vi "SeCrTs-UI Commands_R.vi"(11 "Data FIFO Ref":T1) -> ()   [LabVIEW 2022 SP3]
doc: "Use this template to build a simple state machine design pattern. Each state executes code and determines which state to transition to."
uses:
  RT Controls/SeCrTs-Data FIFO.ctl
  RT Controls/SeCrTs-NS Enum.ctl
  RT Controls/SeCrTs-Data Type Control screen.ctl
  RT Support/SeCrTs-RT_Global_R.vi
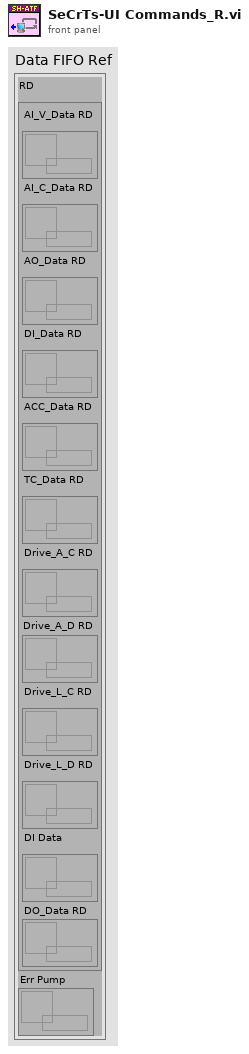
[diagram p1: front panel]
types:
  T1 = typedef "SeCrTs-Data FIFO.ctl" = cluster{"RD":cluster{"AI_V_Data RD":refnum<queue>, "AI_C_Data RD":refnum<queue>, "AO_Data RD":refnum<queue>, "DI_Data RD":refnum<queue>, "ACC_Data RD":refnum<queue>, "TC_Data RD":refnum<queue>, "Drive_A_C RD":refnum<queue>, "Drive_A_D RD":refnum<queue>, "Drive_L_C RD":refnum<queue>, "Drive_L_D RD":refnum<queue>, "DI Data":refnum<queue>, "DO_Data RD":refnum<queue>}, "Err Pump":refnum<queue>}
  T2 = typedef "SeCrTs-Data Type Control screen.ctl" = cluster{"DI_Data":digitalwaveform[], "Drive_A_C":waveform(dbl)[], "Drive_A_D":waveform(dbl)[], "Drive_L_C":waveform(dbl)[], "Drive_L_D":waveform(dbl)[], "Loop Status":bool[], "CDT Timer":dbl, "RT Error":cluster{"Error Code":string, "Error Source":string}, "DO":waveform(dbl)[], "SEQ Monitor":string[], "Device List":string}
  T3 = cluster{"Er":refnum<queue>, "reader":refnum<k21>, "writer ":refnum<k21>}
  T4 = typedef "SeCrTs-NS Enum.ctl" = enum16{"Initialize", "Wait for Connection", "Send data", "Exit"}
  T5 = enum16{"AI C", "AI V", "AO", "DI", "DO", "TC", "ACC", "RT PMP", "DR A"}
  T6 = enum16{"Init", "Read 'All'", "Read 'n'", "Read '1'", "Write '1'", "Write 'n'", "Write 'All'"}
  T7 = cluster{"Start DAQ":bool, "Stop DAQ":bool, "RT Stop":bool, "RT Exit":bool, "Start Seq":bool}
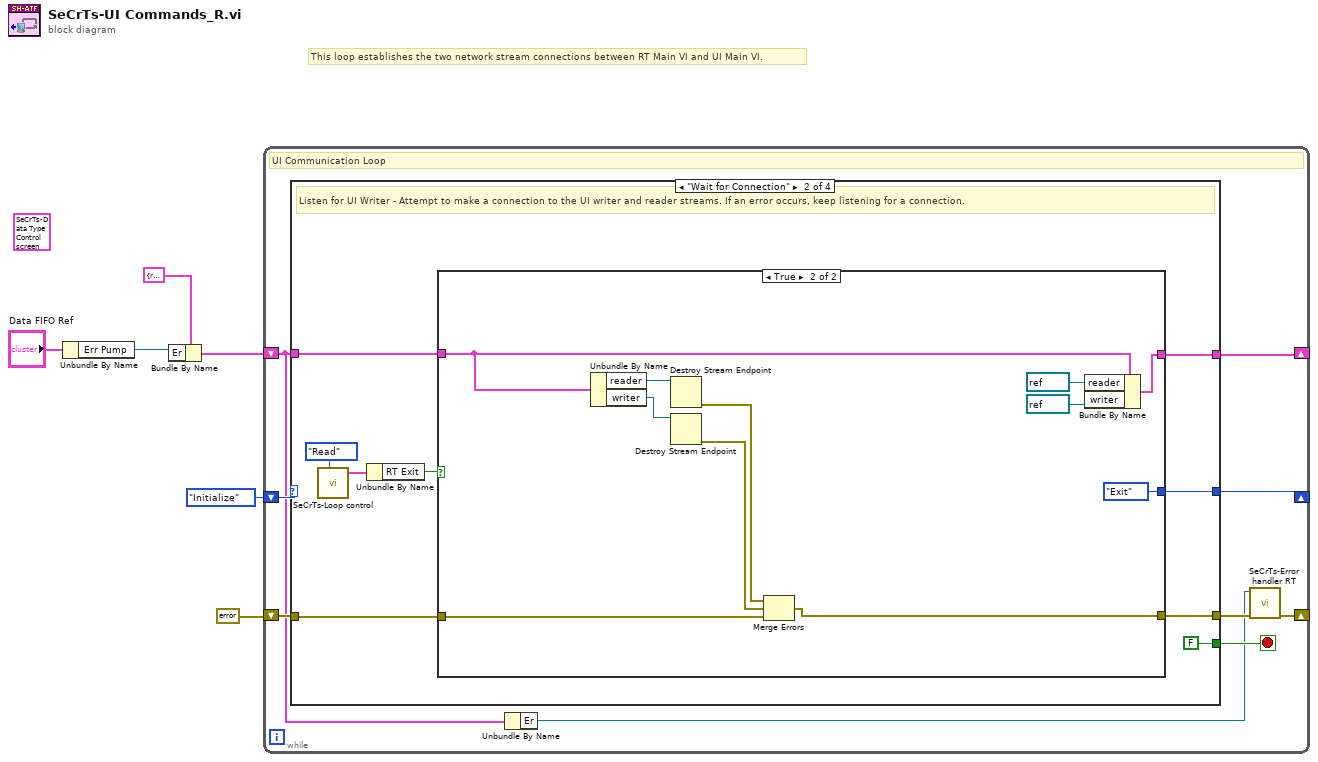
[diagram p0: block diagram]
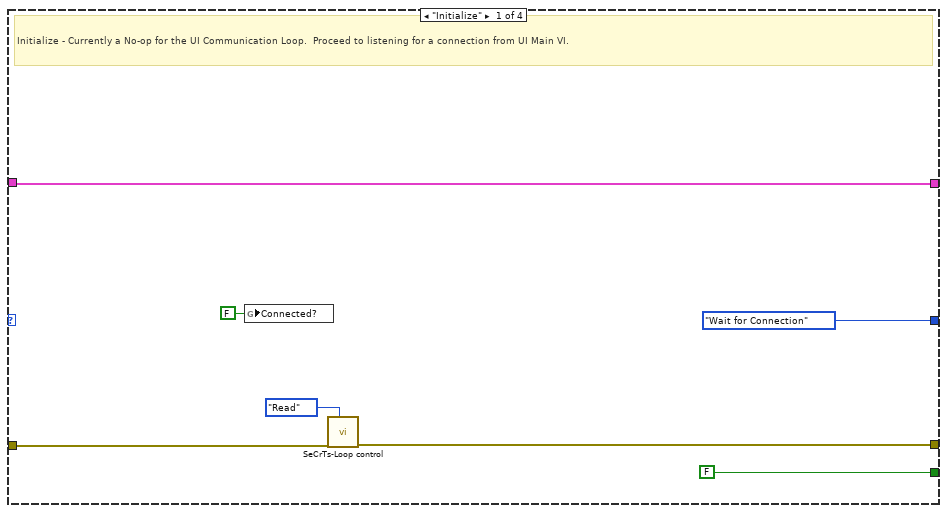
[diagram p2: hidden frame]
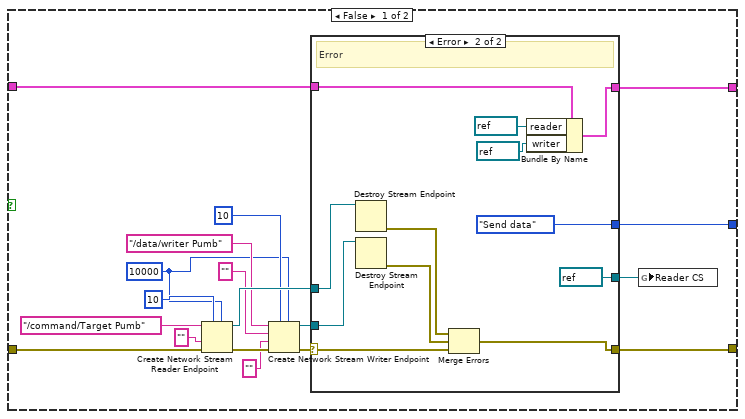
[diagram p3: hidden frame]
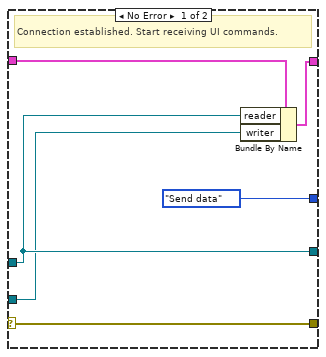
[diagram p4: hidden frame]
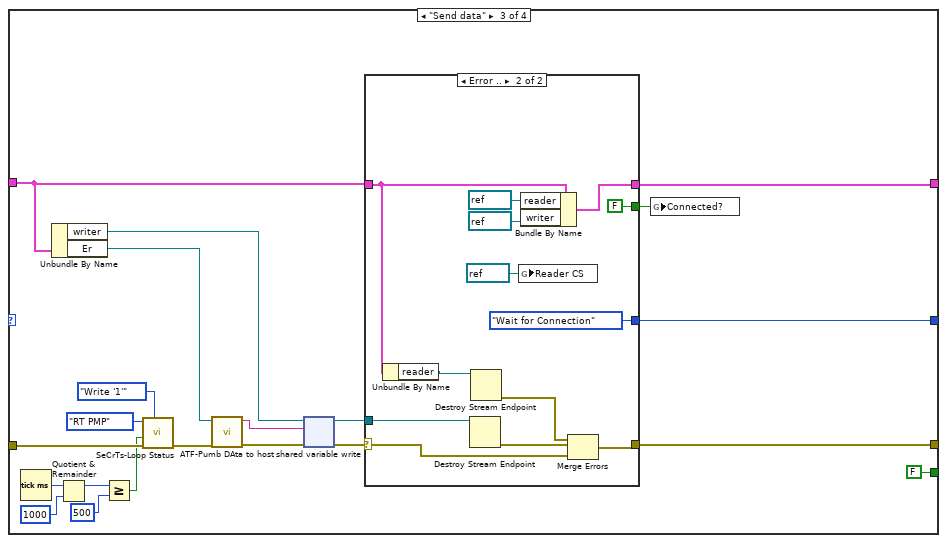
[diagram p5: hidden frame]
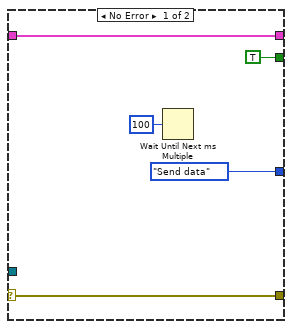
[diagram p6: hidden frame]
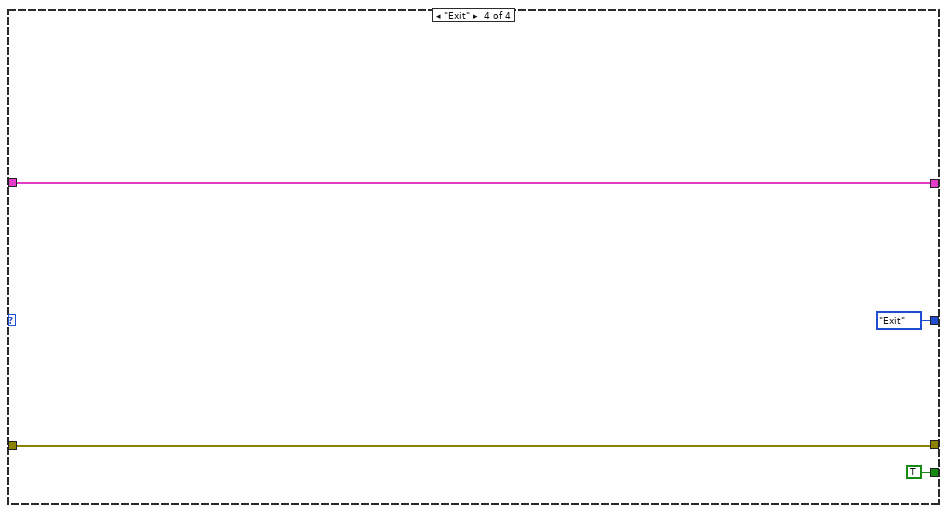
[diagram p7: hidden frame]
diagram:
  (unwired) T2 {"DI_Data"=[], "Drive_A_C"=[], "Drive_A_D"=[], "Drive_L_C"=[], "Drive_L_D"=[], "Loop Status"=[], "CDT Timer"=0.0, "RT Error"={"Error Code"="", "Error Source"=""}, "DO"=[], "SEQ Monitor"=[], "Device List"=""}
  # "This loop establishes the two network stream connections between RT Main VI and UI Main VI."
  n1 = Unbundle By Name("Data FIFO Ref") -> ("Err Pump"=w3:refnum<queue>)
  n2 = Bundle By Name(cluster=T3 {"Er"=refnum, "reader"="", "writer "=""}, "Er"=w3) -> (w2:T3)
  n3 = while {
    shift-right: [w14] -> _
    shift-left: SeCrTs-NS_Enum."Initialize" ("Enum") -> [w15]
    shift-right: [w7] -> _
    shift-left: w2 -> [w9]
    shift-right: [w11] -> _
    shift-left: errorcluster {"status"=FALSE, "code"=0, "source"=""} ("error in (no error)") -> [w10]
    stop <- w12 stop-if-true
    # "UI Communication Loop"
    n4 = case shown="\"Wait for Connection\"" w15 {
      tunnel: [w17 w31 w82 w119] -> w13
      tunnel: [SeCrTs-NS_Enum."Wait for Connection" ("Enum") w30 w83 SeCrTs-NS_Enum."Exit" ("Enum")] -> w14
      tunnel: [FALSE FALSE FALSE TRUE] -> w12
      tunnel: w10 -> [w18 w29 w99 w119]
      tunnel: w9 -> [w16 w28 w85 w121]
      tunnel: [w16 w24 w84 w121] -> w7
      frame "Initialize" {
        # "Initialize - Currently a No-op for the UI Communication Loop.  Proceed to listening for a connection from UI Main VI."
        n5 = global write "SeCrTs-RT_Global_R.vi" "Connected?"(FALSE ("Connected?")) -> ()
        n6 = call "SeCrTs-Loop control.vi"("Action"=enum16{"Init", "Write", "Read"}."Read", "error in (no error)"=w18) -> ("error Out"=w17:errorcluster)  [unwired: 8 in, 1 out]
      }
      frame "Wait for Connection" {
        # "Listen for UI Writer - Attempt to make a connection to the UI writer and reader streams. If an error occurs, keep listening for a connection."
        n7 = call "SeCrTs-Loop control.vi"("Action"=enum16{"Init", "Write", "Read"}."Read") -> ("Loop Control out"=w27:T7)  [unwired: 9 in, 1 out]
        n8 = Unbundle By Name(w27) -> ("RT Exit"=w25:bool)
        n9 = case shown="True" w25 {
          tunnel: [w34 w72] -> w31
          tunnel: [w44 SeCrTs-NS_Enum."Exit" ("Enum")] -> w30
          tunnel: w29 -> [w41 w73]
          tunnel: w28 -> [w37 w71]
          tunnel: [w36 w70] -> w24
          frame False {
            w39 = 10000 ("timeout in ms (-1)")
            n10 = Create Network Stream Reader Endpoint(5:w39, 7:10 ("reader buffer size"), 8:w41, 9:"" ("writer url"), 11:"/command/Target Pumb" ("reader name")) -> (0:w48:errorcluster, 3:w49:refnum<k21>)  [unwired: 2 in]
            n11 = Create Network Stream Writer Endpoint(5:w39, 7:10 ("writer buffer size"), 8:w48, 9:"" ("writer url"), 10:"" ("writer url"), 11:"/data/writer Pumb" ("RT Stream Name_C")) -> (0:w35:errorcluster, 3:w47:refnum<k21>)  [unwired: 1 in]
            n12 = case shown="Error" w35 {
              selector: w35 -> [w50 w57]
              tunnel: w49 -> [w53 w67]
              tunnel: w47 -> [w52 w66]
              tunnel: [w53 refnum<k21> refnum ("reader name")] -> w38
              tunnel: [SeCrTs-NS_Enum."Send data" ("Enum") SeCrTs-NS_Enum."Send data" ("Enum")] -> w44
              tunnel: w37 -> [w54 w63]
              tunnel: [w51 w64] -> w36
              tunnel: [w50 w60] -> w34
              frame No Error {
                # "Connection established. Start receiving UI commands."
                n13 = Bundle By Name(cluster=w54, "reader"=w53, "writer"=w52) -> (w51:T3)
              }
              frame Error {
                # "Error"
                n14 = Destroy Stream Endpoint(11:w67) -> (0:w59:errorcluster)  [unwired: 1 in]
                n15 = Destroy Stream Endpoint(11:w66) -> (0:w58:errorcluster)  [unwired: 1 in]
                n16 = Merge Errors(w59, w58, w57) -> (w60:errorcluster)
                n17 = Bundle By Name(cluster=w63, "reader"=refnum<k21> refnum, "writer"=refnum<k21> refnum) -> (w64:T3)
              }
            }
            n18 = global write "SeCrTs-RT_Global_R.vi" "Reader CS"(w38) -> ()
          }
          frame True {
            n19 = Unbundle By Name(w71) -> ("reader"=w75:refnum<k21>, "writer"=w74:refnum<k21>)
            n20 = Destroy Stream Endpoint(11:w75) -> (0:w77:errorcluster)  [unwired: 1 in]
            n21 = Destroy Stream Endpoint(11:w74) -> (0:w76:errorcluster)  [unwired: 1 in]
            n22 = Merge Errors(w77, w76, w73) -> (w72:errorcluster)
            n23 = Bundle By Name(cluster=w71, "reader"=refnum<k21> refnum, "writer"=refnum<k21> refnum) -> (w70:T3)
          }
        }
      }
      frame "Send data" {
        n24 = Tick Count (ms)() -> (millisecond timer value=w96:u32)
        n25 = Unbundle By Name(w85) -> ("writer"=w89:refnum<k21>, "Er"=w90:refnum<queue>)
        n26 = Quotient & Remainder(x=w96, y=u32 1000) -> (x-y*floor(x/y)=w94:u32)  [unwired: 1 out]
        n27 = Greater Or Equal?(x=w94, y=u32 500) -> (x >= y?=w92:bool)
        n28 = call "SeCrTs-Loop Status.vi"("Option"=T6."Write '1'", "error in (no error)"=w99, "Status"=w92, "Loop"=T5."RT PMP") -> ("error out"=w91:errorcluster)  [unwired: 5 in, 2 out]
        n29 = call "ATF-Pumb DAta to host.vi"("error in (no error)"=w91, "Err"=w90) -> ("error out"=w87:errorcluster, "data"=w88:string)  [unwired: 8 in]
        n30 = shared-variable-write(w89, w87, w88) -> (w80:refnum<k21>, w86:errorcluster)  [unwired: 1 in, 1 out]
        n31 = case shown="Error .." w86 {
          selector: w86 -> [w102 w109]
          tunnel: w85 -> [w104 w112]
          tunnel: [w104 w116] -> w84
          tunnel: [SeCrTs-NS_Enum."Send data" ("Enum") SeCrTs-NS_Enum."Wait for Connection" ("Enum")] -> w83
          tunnel: [w102 w110] -> w82
          tunnel: [TRUE ("Connected?") FALSE ("Connected?")] -> w81
          tunnel: w80 -> [_ w113]
          frame No Error {
            n32 = Wait Until Next ms Multiple(millisecond multiple=u32 100) -> ()  [unwired: 1 out]
          }
          frame Error {
            n33 = Unbundle By Name(w112) -> ("reader"=w111:refnum<k21>)
            n34 = Destroy Stream Endpoint(11:w113) -> (0:w108:errorcluster)  [unwired: 1 in]
            n35 = Destroy Stream Endpoint(11:w111) -> (0:w107:errorcluster)  [unwired: 1 in]
            n36 = global write "SeCrTs-RT_Global_R.vi" "Reader CS"(refnum<k21> refnum ("Reader CS")) -> ()
            n37 = Bundle By Name(cluster=w112, "reader"=refnum<k21> refnum, "writer"=refnum<k21> refnum) -> (w116:T3)
            n38 = Merge Errors(w107, w108, w109) -> (w110:errorcluster)
          }
        }
        n39 = global write "SeCrTs-RT_Global_R.vi" "Connected?"(w81) -> ()
      }
      frame "Exit" {
      }
    }
    n40 = Unbundle By Name(w9) -> ("Er"=w8:refnum<queue>)
    n41 = call "SeCrTs-Error handler RT.vi"("error in"=w13, "Message Queue"=w8) -> ("error out"=w11:errorcluster)  [unwired: 8 in, 1 out]
  }
